vi "Show Image Source Settings.vi"(8 "error in (no error)":errorcluster, 11 "AF IMAQ Display in":refnum<class "HIJ IMAQdx Display.lvclass">) -> (0 "error out":errorcluster, 3 "AF IMAQ Display out":refnum<class "HIJ IMAQdx Display.lvclass">)   [LabVIEW 2014, in "HIJ IMAQdx Display.lvlib" / "HIJ IMAQdx Display.lvclass"]
uses:
  HIJ IMAQdx Display.lvclass
  HIJ Vision Display/HIJ Vision Display/HIJ Vision Display.lvclass/HIJ Vision Display.ctl
  <vilib>/ActorFramework/Message Enqueuer/Message Enqueuer.lvclass/Message Enqueuer.ctl
  HIJ Vision Display/HIJ Vision Display/Read Image Source.vi
  <vilib>/ActorFramework/Message Enqueuer/Enqueue.vi
  <vilib>/ActorFramework/Message Priority Queue/Priority Enqueue.vi
  <vilib>/ActorFramework/Message Enqueuer/Message Enqueuer.lvclass
  Camera Actors/Camera Actor/Camera Actor Messages/open camera settings Msg/open camera settings Msg.lvclass
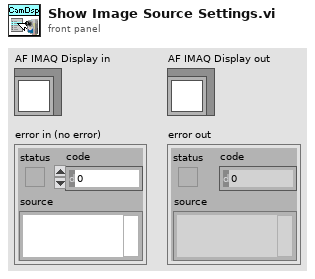
[diagram p1: front panel]
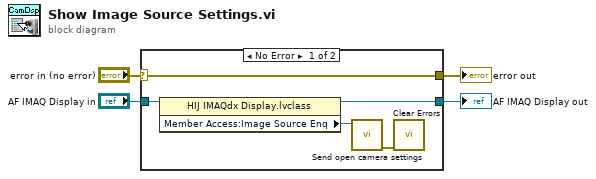
[diagram p0: block diagram]
diagram:
  n1 = case shown="No Error" "error in (no error)" {
    selector: "error in (no error)" -> [w9 w11]
    tunnel: [w9 w11] -> w3
    tunnel: [w6 w10] -> w1
    tunnel: "AF IMAQ Display in" -> [w8 w10]
    frame No Error {
      n2 = property class="HIJ IMAQdx Display.lvclass"(reference=w8) -> (reference out=w6:refnum<class "HIJ IMAQdx Display.lvclass">, "Member Access:Image Source Enq"=w5:refnum<class "Message Enqueuer.lvclass">)  [unwired: 1 in, 1 out]
      n3 = call "Send open camera settings.vi"("Message Enqueuer"=w5) -> ("error out"=w7:errorcluster)  [unwired: 9 in, 1 out]
      n4 = call <vilib>:"Clear Errors.vi"("error in (no error)"=w7) -> ()  [unwired: 5 in, 2 out]
    }
    frame Error {
    }
  }
  "error out" <- w3
  "AF IMAQ Display out" <- w1
